vi "timeset (SubVI).vi"(11 "data":waveform(dbl)[](array[waveform])) -> (3 "Numeric":dbl)   [LabVIEW 2019]
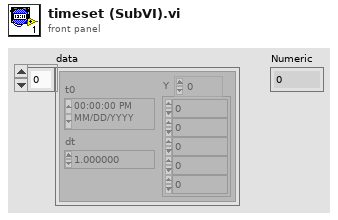
[diagram p1: front panel]
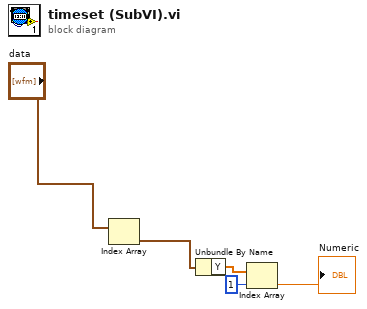
[diagram p0: block diagram]
diagram:
  n1 = Index Array(array="data") -> (element=w2:waveform(dbl))  [unwired: 1 in]
  n2 = Unbundle By Name(w2) -> ("Y"=w3:dbl[])
  n3 = Index Array(array=w3, index=1) -> (element=→"Numeric":dbl)
